vi "convert manual string to nufern response string.vi"(8 "error in (no error)":errorcluster, 11 "Manual String":string) -> (0 "error out":errorcluster, 3 "result string":string)   [LabVIEW 2016]
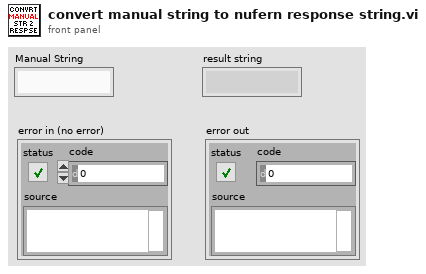
[diagram p1: front panel]
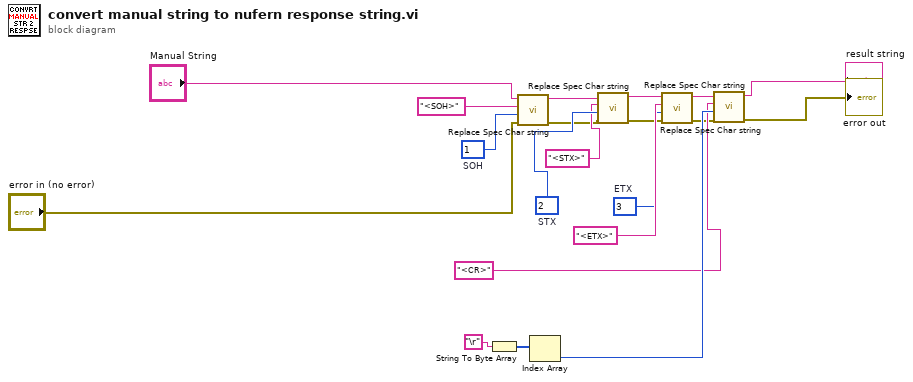
[diagram p0: block diagram]
diagram:
  w9 = 3  # ETX
  w8 = 2  # STX
  w3 = 1  # SOH
  n1 = String To Byte Array(string="\r") -> (unsigned byte array=w19:u8[])
  n2 = call "Replace Spec Char string.vi"("error in (no error)"="error in (no error)", "SOH"=w3, "search string"="<SOH>", "String"="Manual String") -> ("error out"=w5:errorcluster, "result string"=w6:string)  [unwired: 6 in]
  n3 = Index Array(array=w19) -> (element=w20:u8)  [unwired: 1 in]
  n4 = call "Replace Spec Char string.vi"("error in (no error)"=w5, "SOH"=w8, "search string"="<STX>", "String"=w6) -> ("error out"=w11:errorcluster, "result string"=w10:string)  [unwired: 6 in]
  n5 = call "Replace Spec Char string.vi"("error in (no error)"=w11, "SOH"=w9, "search string"="<ETX>", "String"=w10) -> ("error out"=w13:errorcluster, "result string"=w14:string)  [unwired: 6 in]
  n6 = call "Replace Spec Char string.vi"("error in (no error)"=w13, "SOH"=w20, "search string"="<CR>", "String"=w14) -> ("error out"=→"error out":errorcluster, "result string"=→"result string":string)  [unwired: 6 in]
